vi "main.vi"() -> ()   [LabVIEW 2018]
uses:
  <vilib>/httpClient/ClientHandle.ctl
  <vilib>/httpClient/PUTBuffer.vi
  <vilib>/httpClient/LabVIEWHTTPClient.lvlib
panel:
  out "EntitiesList":string[](array[string])
  in  "Update":bool
  in  "Delete":bool
  in  "Show":bool
  in  "Create":bool
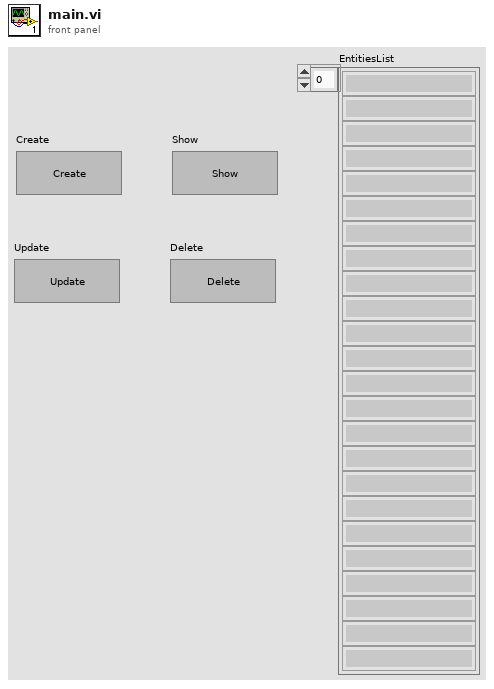
[diagram p1: front panel]
types:
  T1 = typedef "LabVIEWHTTPClient.lvlib/ClientHandle.ctl" = refnum<k1>
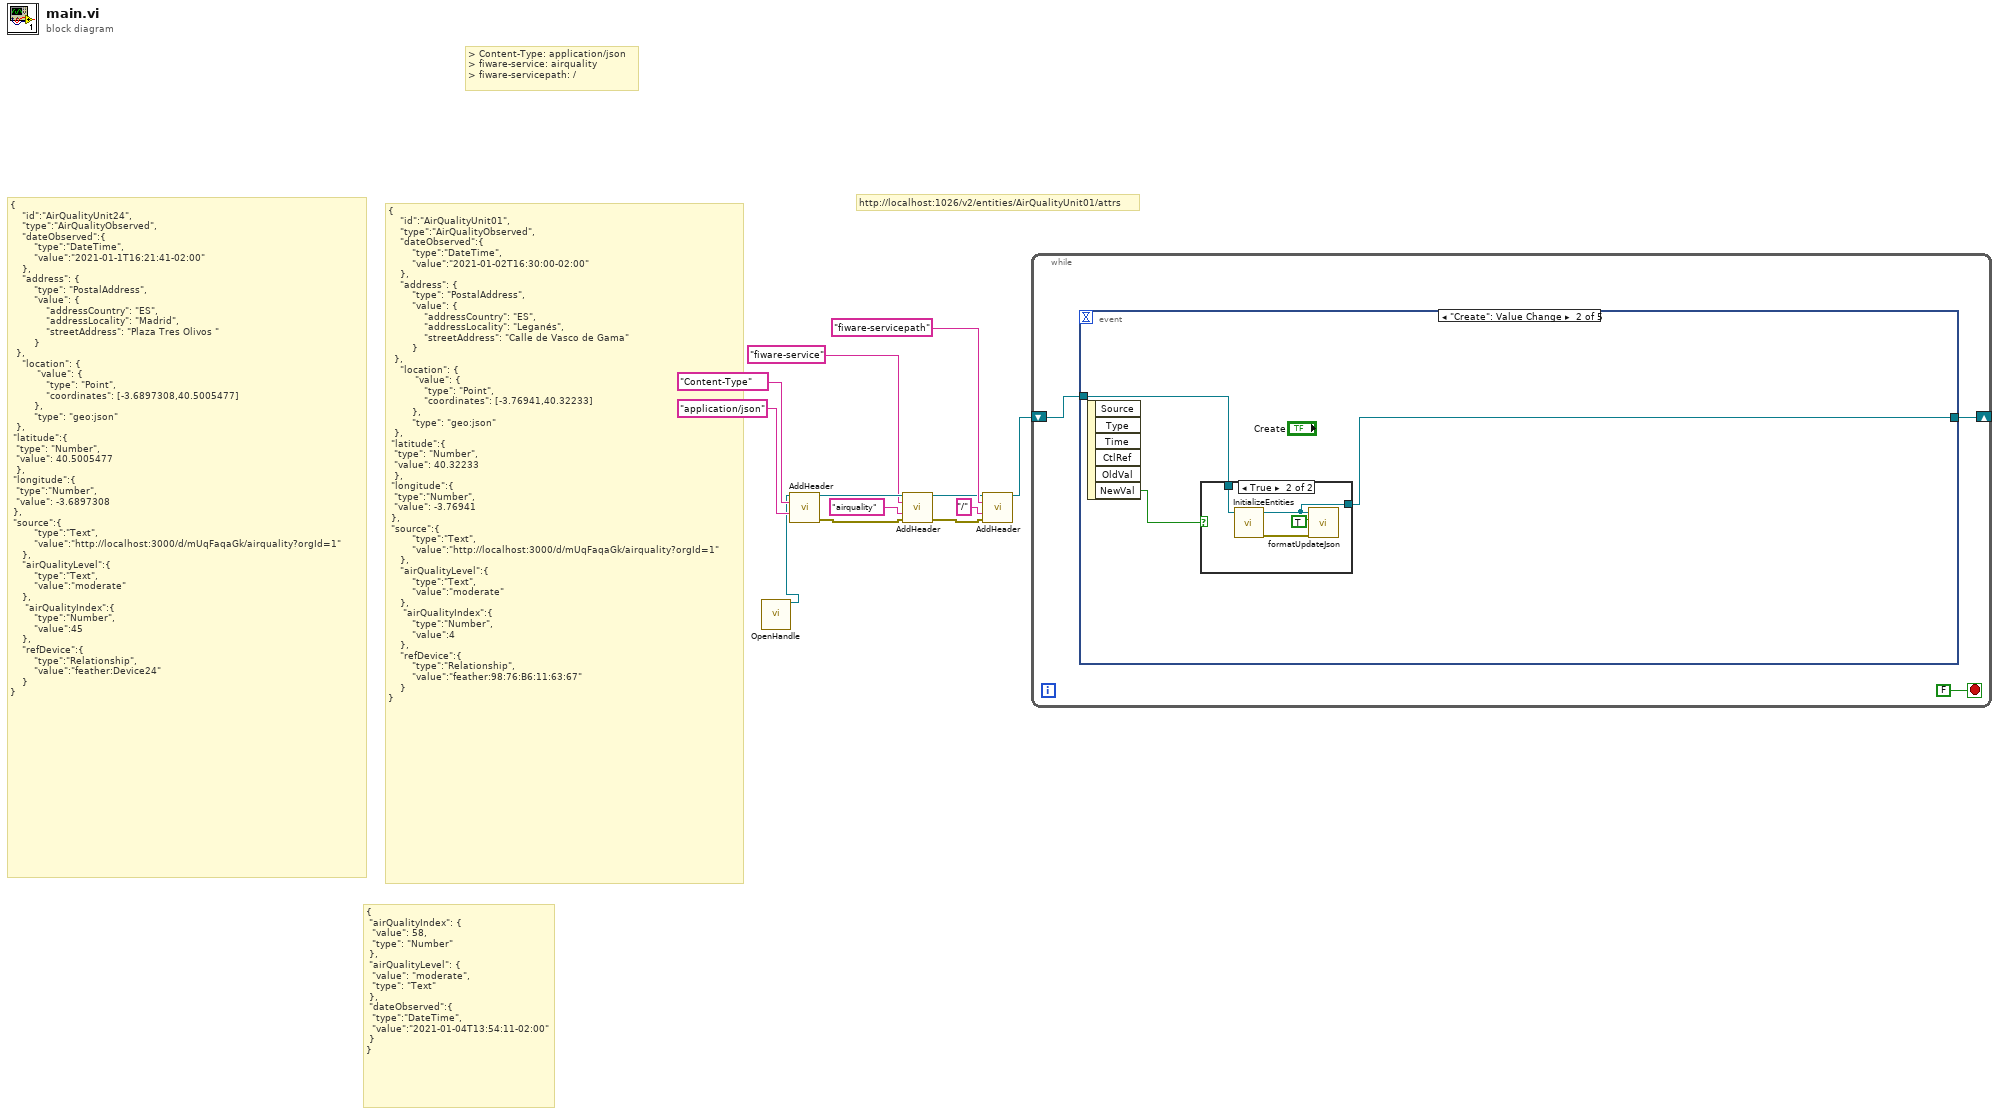
[diagram p0: block diagram]
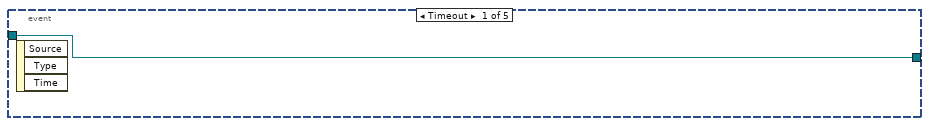
[diagram p2: hidden frame]
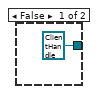
[diagram p3: hidden frame]
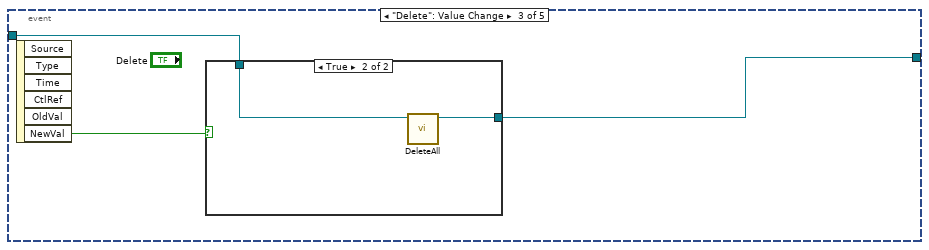
[diagram p4: hidden frame]
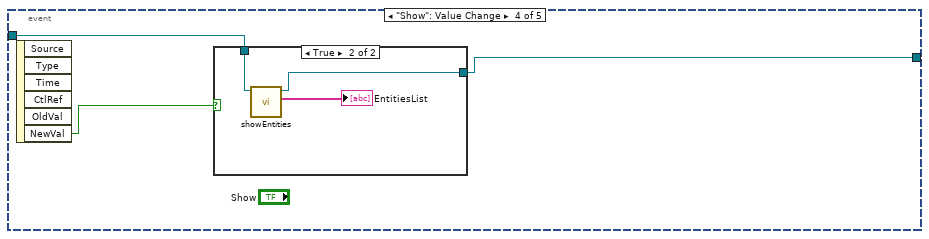
[diagram p6: hidden frame]
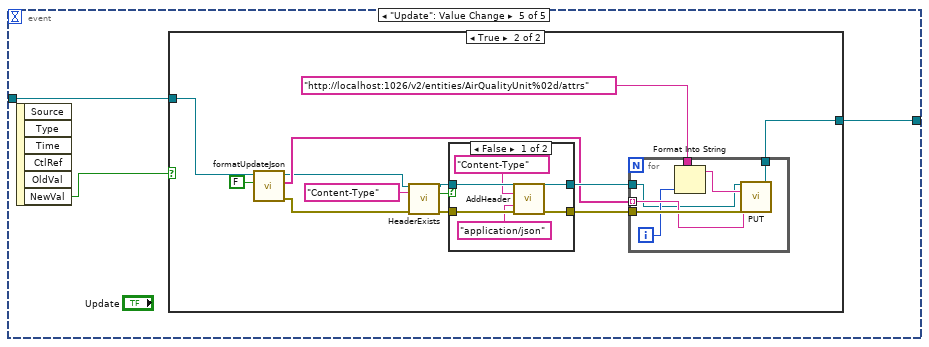
[diagram p8: hidden frame]
diagram:
  # "http://localhost:1026/v2/entities/AirQualityUnit01/attrs"
  # "{\n\t\"airQualityIndex\": {\n\t\t\"value\": 58,\n\t\t\"type\": \"Number\"\n\t},\n\t\"airQualityLevel\": {\n\t\t\"value\": \"moderate\",\n\t\t\"type\": \"Text\"\n\t},\n\t\"dateObserved\":{\n\t\t\"type\":\"DateTime\",\n\t\t\"value\":\"2021-01-04T13:54:11-02:00\"\n\t}\n}"
  # "{\n    \"id\":\"AirQualityUnit24\",\n    \"type\":\"AirQualityObserved\",\n    \"dateObserved\":{\n        \"type\":\"DateTime\",\n        \"value\":\"2021-01-1T16:21:41-02:00\"\n    },\n    \"address\": {\n        \"type\": \"PostalAddress\",\n        \"value\": {\n            \"addressCountry\": \"ES\",\n            \"addressLocality\": \"Madrid\",\n            \"streetAddress\": \"Plaza Tres Olivos \"           \n        }\n\t\t},\n    \"location\": {\n         \"value\": {\n            \"type\": \"Point\",\n            \"coordinates\": [-3.6897308,40.5005477]\n        },\n        \"type\": \"geo:json\"\n  },\n\t\"latitude\":{\n\t\t\"type\": \"Number\",\n\t\t\"value\": 40.5005477\n\t\t},\n\t\"longitude\":{\n\t\t\"type\":\"Number\",\n\t\t\"value\": -3.6897308\n\t},\n\t\"source\":{\n        \"type\":\"Text\",\n        \"value\":\"http://localhost:3000/d/mUqFaqaGk/airquality?orgId=1\"\n    },\n    \"airQualityLevel\":{\n        \"type\":\"Text\",\n        \"value\":\"moderate\"\n    },\n\t    \"airQualityIndex\":{\n        \"type\":\"Number\",\n        \"value\":45\n    },\n    \"refDevice\":{\n        \"type\":\"Relationship\",\n        \"value\":\"feather:Device24\"\n    }\n}"
  # "> Content-Type: application/json\n> fiware-service: airquality\n> fiware-servicepath: /"
  # "{\n    \"id\":\"AirQualityUnit01\",\n    \"type\":\"AirQualityObserved\",\n    \"dateObserved\":{\n        \"type\":\"DateTime\",\n        \"value\":\"2021-01-02T16:30:00-02:00\"\n    },\n    \"address\": {\n        \"type\": \"PostalAddress\",\n        \"value\": {\n            \"addressCountry\": \"ES\",\n            \"addressLocality\": \"Leganés\",\n            \"streetAddress\": \"Calle de Vasco de Gama\"           \n        }\n\t\t},\n    \"location\": {\n         \"value\": {\n            \"type\": \"Point\",\n            \"coordinates\": [-3.76941,40.32233]\n        },\n        \"type\": \"geo:json\"\n  },\n\t\"latitude\":{\n\t\t\"type\": \"Number\",\n\t\t\"value\": 40.32233\n\t\t},\n\t\"longitude\":{\n\t\t\"type\":\"Number\",\n\t\t\"value\": -3.76941\n\t},\n\t\"source\":{\n        \"type\":\"Text\",\n        \"value\":\"http://localhost:3000/d/mUqFaqaGk/airquality?orgId=1\"\n    },\n    \"airQualityLevel\":{\n        \"type\":\"Text\",\n        \"value\":\"moderate\"\n    },\n\t    \"airQualityIndex\":{\n        \"type\":\"Number\",\n        \"value\":4\n    },\n    \"refDevice\":{\n        \"type\":\"Relationship\",\n        \"value\":\"feather:98:76:B6:11:63:67\"\n    }\n}"
  n1 = call <vilib>:"OpenHandle.vi"() -> ("client handle out"=w2:T1)  [unwired: 14 in, 1 out]
  n2 = call <vilib>:"AddHeader.vi"("client handle"=w2, "header"="Content-Type", "value"="application/json") -> ("client handle out"=w12:T1, "error out"=w6:errorcluster)  [unwired: 11 in]
  n3 = call <vilib>:"AddHeader.vi"("client handle"=w12, "header"="fiware-service" ("value"), "value"="airquality", "error in (no error)"=w6) -> ("client handle out"=w8:T1, "error out"=w4:errorcluster)  [unwired: 10 in]
  n4 = call <vilib>:"AddHeader.vi"("client handle"=w8, "header"="fiware-servicepath" ("value"), "value"="/", "error in (no error)"=w4) -> ("client handle out"=w1:T1)  [unwired: 10 in, 1 out]
  n5 = while {
    shift-right: [w14] -> _
    shift-left: w1 -> [w13]
    stop <- FALSE stop-if-true
    n6 = event shown="[1] \"Create\": Value Change" {
      selector: _ -> [_ _ _ _ _]
      dyn-events: _ -> [_ _ _ _ _]
      timeout: _ -> [_ _ _ _ _]
      tunnel: [w16 w18 w25 w31 w38] -> w14
      tunnel: w13 -> [w16 w17 w26 w32 w39]
      event Timeout {
        n7 = event-data() -> ()  [unwired: 1 in, 3 out]
      }
      event "Create": Value Change {
        n8 = event-data() -> ("NewVal"=w19:bool)  [unwired: 1 in, 5 out]
        n9 = case shown="True" w19 {
          tunnel: [T1 refnum ("Refnum out") w23] -> w18
          tunnel: w17 -> [_ w21]
          frame False {
          }
          frame True {
            n10 = call "InitializeEntities.vi"("client handle"=w21) -> ("error out"=w24:errorcluster, "Refnum out"=w23:T1)  [unwired: 9 in]
            n11 = call "formatUpdateJson.vi"("error in (no error)"=w24, "Init/Update"=TRUE, "Refnum in"=w23) -> ()  [unwired: 6 in, 3 out]
          }
        }
      }
      event "Delete": Value Change {
        n12 = event-data() -> ("NewVal"=w27:bool)  [unwired: 1 in, 5 out]
        n13 = case shown="True" w27 {
          tunnel: w26 -> [w28 w30]
          tunnel: [w28 w29] -> w25
          frame False {
          }
          frame True {
            n14 = call "DeleteAll.vi"("Refnum in"=w30) -> ("Refnum out"=w29:T1)  [unwired: 9 in, 1 out]
          }
        }
      }
      event "Show": Value Change {
        n15 = event-data() -> ("NewVal"=w33:bool)  [unwired: 1 in, 5 out]
        n16 = case shown="True" w33 {
          tunnel: w32 -> [w34 w36]
          tunnel: [w34 w35] -> w31
          frame False {
          }
          frame True {
            n17 = call "showEntities.vi"("Refnum in"=w36) -> ("EntitiesList"=→"EntitiesList":string[], "Refnum out"=w35:T1)  [unwired: 8 in, 1 out]
          }
        }
      }
      event "Update": Value Change {
        n18 = event-data() -> ("NewVal"=w40:bool)  [unwired: 1 in, 5 out]
        n19 = case shown="True" w40 {
          tunnel: w39 -> [w41 w45]
          tunnel: [w41 w46] -> w38
          frame False {
          }
          frame True {
            n20 = call "formatUpdateJson.vi"("Init/Update"=FALSE, "Refnum in"=w45) -> ("error out"=w49:errorcluster, "Update Data"=w47:string[], "Refnum out"=w43:T1)  [unwired: 7 in]
            n21 = call <vilib>:"HeaderExists.vi"("client handle"=w43, "header"="Content-Type", "error in (no error)"=w49) -> ("client handle out"=w53:T1, "header exists?"=w48:bool, "error out"=w54:errorcluster)  [unwired: 9 in, 1 out]
            n22 = case shown="False" w48 {
              tunnel: w54 -> [w67 w68]
              tunnel: w53 -> [w66 w69]
              tunnel: [w65 w68] -> w52
              tunnel: [w64 w69] -> w51
              frame False {
                n23 = call <vilib>:"AddHeader.vi"("client handle"=w66, "header"="Content-Type", "value"="application/json", "error in (no error)"=w67) -> ("client handle out"=w64:T1, "error out"=w65:errorcluster)  [unwired: 10 in]
              }
              frame True {
              }
            }
            n24 = for {
              tunnel: w52 -> [w61]
              tunnel: w51 -> [w55]
              tunnel: w47 -> [w60] mode=indexing
              tunnel: [w59] -> w46
              tunnel: "http://localhost:1026/v2/entities/AirQualityUnit%02d/attrs" -> [w58]
              i -> [w57]
              n25 = Format Into String(format string=w58, w57) -> (resulting string=w56:string)  [unwired: 2 in, 1 out]
              n26 = call-poly <vilib>:"PUT.vi"("client handle"=w55, "url"=w56, "buffer"=w60, "error in (no error)"=w61) -> ("client handle out"=w59:T1)  [unwired: 8 in, 3 out]
            }
          }
        }
      }
    }
  }
